vi "get_rumble_video_data.vi"(0 "HTTP client handle":T1, 1 "Private IDs (F)":bool, 3 "Embed delta":refnum<queue>, 5 "Video ID":cluster{"Index":i32, "Canonical ID":i32}, 7 "Thumbnails folder":path, 11 "error in (no error)":errorcluster, 12 "Rate limit ref.":refnum<vi>, 14 "Result queue":refnum<queue>) -> (4 "client handle out":T1, 15 "error out":errorcluster)   [LabVIEW 2023]
uses:
  <vilib>/httpClient/ClientHandle.ctl
  <vilib>/httpClient/LabVIEWHTTPClient.lvlib
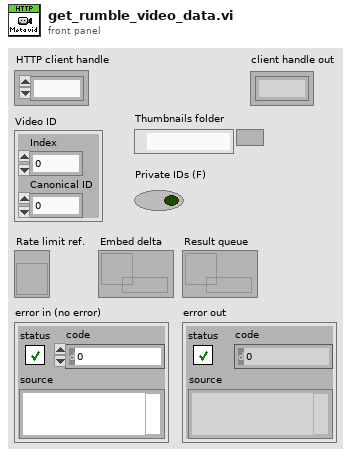
[diagram p1: front panel]
types:
  T1 = typedef "LabVIEWHTTPClient.lvlib/ClientHandle.ctl" = refnum<k1>
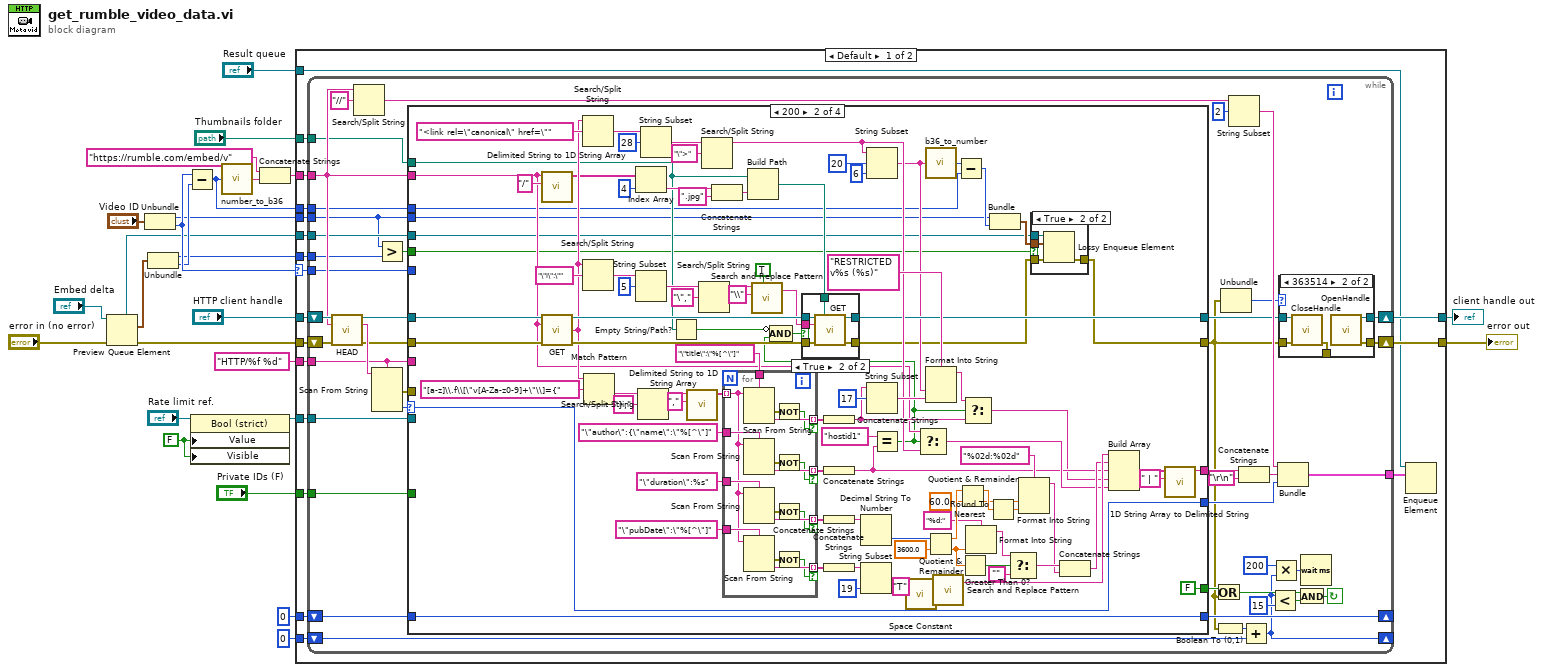
[diagram p0: block diagram]
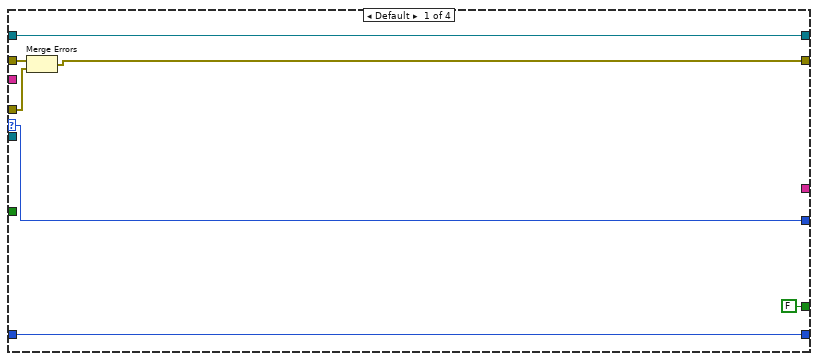
[diagram p3: hidden frame]
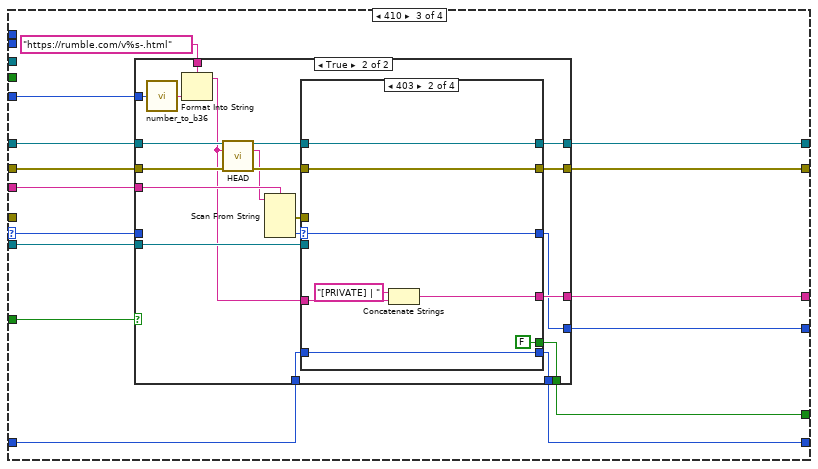
[diagram p6: hidden frame]
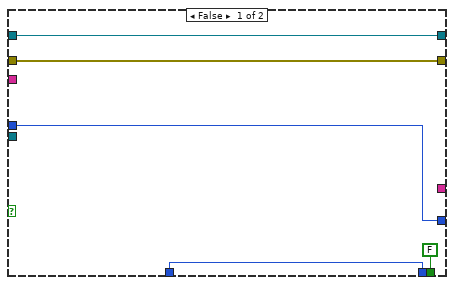
[diagram p7: hidden frame]
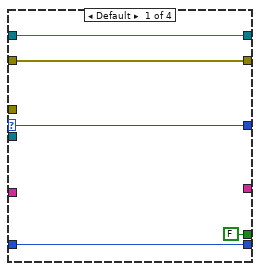
[diagram p8: hidden frame]
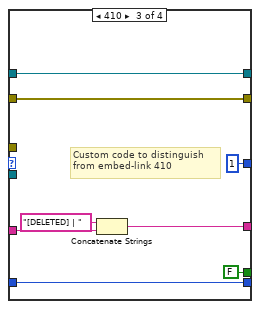
[diagram p9: hidden frame]
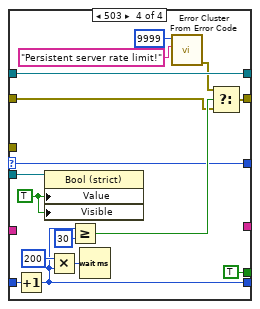
[diagram p10: hidden frame]
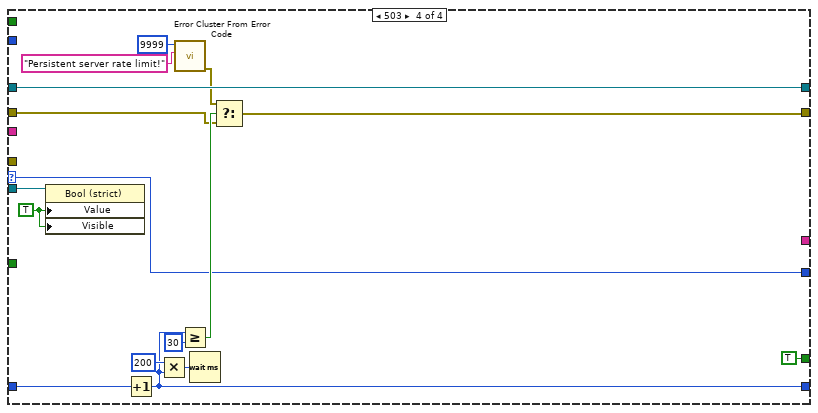
[diagram p11: hidden frame]
diagram:
  w18 = FALSE ("Value")
  n1 = Preview Queue Element(queue="Embed delta", error in (no error)="error in (no error)") -> (queue out=w4:refnum<queue>, element=w9:cluster{"Index":i32, "Embed delta":i32}, error out=w8:errorcluster)  [unwired: 1 in, 1 out]
  n2 = Unbundle("Video ID") -> ("Index"=w1:i32, "Canonical ID"=w7:i32)
  n3 = Unbundle(w9) -> ("Index"=w3:i32, "Embed delta"=w6:i32)
  n4 = Subtract(x=w7, y=w6) -> (x-y=w2:i32)
  n5 = property class="Bool (strict)"(reference="Rate limit ref.", "Value"=w18, "Visible"=w18) -> (reference out=w21:refnum<vi>)  [unwired: 1 in, 1 out]
  n6 = call "number_to_b36.vi"("Number"=w2) -> ("Base36 string"=w5:string)
  n7 = Concatenate Strings("https://rumble.com/embed/v" ("url"), w5) -> (w14:string)
  n8 = case shown="Default" w7 {
    selector: w7 -> [w31 _]
    tunnel: [w44 w324] -> w26
    tunnel: [w43 w323] -> w25
    tunnel: "HTTP client handle" -> [w42 w324]
    tunnel: w8 -> [w41 w323]
    tunnel: "HTTP/%f %d" ("format string") -> [w40 _]
    tunnel: w21 -> [w39 _]
    tunnel: 0 -> [w38 _]
    tunnel: 0 -> [w37 _]
    tunnel: w14 -> [w35 _]
    tunnel: "Thumbnails folder" -> [w34 _]
    tunnel: "Result queue" -> [w33 _]
    tunnel: "Private IDs (F)" -> [w32 _]
    tunnel: w4 -> [w30 _]
    tunnel: w1 -> [w29 _]
    tunnel: w3 -> [w28 _]
    tunnel: w2 -> [w27 _]
    frame Default {
      n9 = while {
        tunnel: w40 -> [w63]
        tunnel: w39 -> [w84]
        shift-right: [w52] -> w44
        shift-left: w42 -> [w88]
        shift-right: [w51] -> w43
        shift-left: w41 -> [w87]
        shift-right: [w59] -> _
        shift-left: w38 -> [w82]
        shift-right: [w79] -> _
        shift-left: w37 -> [w80]
        tunnel: w35 -> [w69]
        tunnel: [w70] -> w36
        tunnel: w34 -> [w65]
        tunnel: w31 -> [w64]
        tunnel: w32 -> [w50]
        tunnel: w30 -> [w49]
        tunnel: w29 -> [w48]
        tunnel: w28 -> [w46]
        tunnel: w27 -> [w47]
        stop <- w75 continue-if-true
        n10 = call <vilib>:"HEAD.vi"("client handle"=w88, "url"=w69, "error in (no error)"=w87) -> ("client handle out"=w85:T1, "headers"=w86:string, "error out"=w57:errorcluster)  [unwired: 10 in]
        n11 = Search/Split String(string=w69, search string/char (-)="//") -> (match + rest of string=w67:string)  [unwired: 1 in, 2 out]
        n12 = Scan From String(format string=w63, input string=w86) -> (error out=w72:errorcluster, output 2=w58:i32)  [unwired: 5 in, 2 out]
        n13 = Greater?(x=w48, y=w46) -> (0:w45:bool)
        n14 = case shown="200" w58 {
          selector: w58 -> [w96 w113 w234 w307]
          tunnel: [w102 w136 w240 w322] -> w54
          tunnel: [w97 w104 w239 w309] -> w53
          tunnel: w85 -> [w102 w152 w244 w322]
          tunnel: w57 -> [w99 w151 w243 w311]
          tunnel: w69 -> [_ w119 _ _]
          tunnel: [_ w155 w231 _] -> w73
          tunnel: w84 -> [_ _ w241 w321]
          tunnel: [FALSE FALSE w235 TRUE] -> w81
          tunnel: w80 -> [w100 w153 w238 w319]
          tunnel: [w100 w153 w237 w315] -> w79
          tunnel: w72 -> [w98 _ _ _]
          tunnel: w65 -> [_ w117 _ _]
          tunnel: w64 -> [_ _ w230 _]
          tunnel: w63 -> [_ _ w242 _]
          tunnel: [w96 w113 w236 w307] -> w62
          tunnel: w50 -> [_ _ w233 _]
          tunnel: w49 -> [_ w106 _ _]
          tunnel: w48 -> [_ w108 _ _]
          tunnel: w47 -> [_ w110 _ _]
          tunnel: w45 -> [_ w103 _ _]
          frame Default {
            n15 = Merge Errors(w99, w98) -> (w97:errorcluster)
          }
          frame 200 {
            n16 = call <vilib>:"Delimited String to 1D String Array.vi"("delimiter"="/", "delimited string"=w119) -> ("string array"=w124:string[])  [unwired: 9 in]
            n17 = call <vilib>:"GET.vi"("client handle"=w152, "url"=w119, "error in (no error)"=w151) -> ("client handle out"=w138:T1, "body"=w127:string, "error out"=w137:errorcluster)  [unwired: 9 in, 1 out]
            n18 = Search/Split String(string=w127, search string/char (-)="<link rel=\"canonical\" href=\"") -> (match + rest of string=w165:string)  [unwired: 1 in, 2 out]
            n19 = Search/Split String(string=w127, search string/char (-)="\"i\":\"") -> (match + rest of string=w129:string)  [unwired: 1 in, 2 out]
            n20 = Match Pattern(string=w127, regular expression="[a-z]\\.f\\[\"v[A-Za-z0-9]+\"\\]={") -> (after substring=w197:string)  [unwired: 1 in, 3 out]
            n21 = Index Array(array=w124, index=4) -> (element=w120:string)
            n22 = String Subset(string=w129, offset (0)=5) -> (substring=w132:string)  [unwired: 1 in]
            n23 = Search/Split String(string=w197, search string/char (-)="};") -> (substring before match=w196:string)  [unwired: 1 in, 2 out]
            n24 = String Subset(string=w165, offset (0)=28 ("y")) -> (substring=w168:string)  [unwired: 1 in]
            n25 = Empty String/Path?(string/path=w117) -> (empty?=w116:bool)
            n26 = call <vilib>:"Delimited String to 1D String Array.vi"("delimiter"=",", "delimited string"=w196) -> ("string array"=w194:string[])  [unwired: 9 in]
            n27 = Search/Split String(string=w132, search string/char (-)="\",") -> (substring before match=w133:string)  [unwired: 1 in, 2 out]
            n28 = Search/Split String(string=w168, search string/char (-)="\">") -> (substring before match=w139:string)  [unwired: 1 in, 2 out]
            n29 = Concatenate Strings(w120, ".jpg" ("string")) -> (w121:string)
            n30 = for {
              tunnel: w194 -> [w213] mode=indexing
              tunnel: "\"title\":\"%[^\"]" ("String") -> [w229]
              tunnel: "\"author\":{\"name\":\"%[^\"]" ("String") -> [w228]
              tunnel: "\"duration\":%s" ("String") -> [w227]
              tunnel: "\"pubDate\":\"%[^\"]" ("String") -> [w226]
              tunnel: [w225] -> w189 mode=indexing if=w217
              tunnel: [w224] -> w188 mode=indexing if=w216
              tunnel: [w223] -> w187 mode=indexing if=w215
              tunnel: [w222] -> w186 mode=indexing if=w214
              n31 = Scan From String(format string=w229, input string=w213) -> (error out=w221:errorcluster, output 1=w225:string)  [unwired: 3 in, 2 out]
              n32 = Scan From String(format string=w228, input string=w213) -> (error out=w220:errorcluster, output 1=w224:string)  [unwired: 3 in, 2 out]
              n33 = Scan From String(format string=w227, input string=w213) -> (error out=w219:errorcluster, output 1=w223:string)  [unwired: 3 in, 2 out]
              n34 = Scan From String(format string=w226, input string=w213) -> (error out=w218:errorcluster, output 1=w222:string)  [unwired: 3 in, 2 out]
              n35 = Not(x=w221) -> (.not. x?=w217:bool)
              n36 = Not(x=w220) -> (.not. x?=w216:bool)
              n37 = Not(x=w219) -> (.not. x?=w215:bool)
              n38 = Not(x=w218) -> (.not. x?=w214:bool)
            }
            n39 = Build Path(base path=w117, name or relative path=w121) -> (appended path=w118:path)
            n40 = call <vilib>:"Search and Replace Pattern.vi"("string"=w133, "regular expression (\"\")"="\\" ("regular expression (\"\")"), "replace all? (F)"=TRUE) -> ("result string"=w126:string)  [unwired: 2 in, 1 out]
            n41 = Concatenate Strings(w189) -> (w143:string)
            n42 = Concatenate Strings(w188) -> (w148:string)
            n43 = Concatenate Strings(w187) -> (w185:string)
            n44 = Concatenate Strings(w186) -> (w164:string)
            n45 = Decimal String To Number(string=w185) -> (number=w170:i32)  [unwired: 2 in, 1 out]
            n46 = String Subset(string=w164, length (rest)=19 ("length (rest)")) -> (substring=w162:string)  [unwired: 1 in]
            n47 = String Subset(string=w139, offset (0)=20 ("y"), length (rest)=6 ("length (rest)")) -> (substring=w112:string)
            n48 = String Subset(string=w143, offset (0)=17 ("y")) -> (substring=w145:string)  [unwired: 1 in]
            n49 = Equal?(x="hostid1", y=w148) -> (x = y?=w114:bool)
            n50 = Compound Arithmetic op=AND(invert w116, w114) -> (w115:bool)
            n51 = case shown="True" w115 {
              tunnel: w138 -> [w206 w212]
              tunnel: w137 -> [w205 w211]
              tunnel: [w206 w210] -> w136
              tunnel: [w205 w209] -> w105
              tunnel: w126 -> [_ w208]
              tunnel: w118 -> [_ w207]
              frame False {
              }
              frame True {
                n52 = call <vilib>:"GET.vi"("client handle"=w212, "output file"=w207, "url"=w208, "error in (no error)"=w211) -> ("client handle out"=w210:T1, "error out"=w209:errorcluster)  [unwired: 8 in, 2 out]
              }
            }
            n53 = call <vilib>:"Space Constant.vi"() -> ("String"=w160:string)
            n54 = Select(t=w119, s=w114, f=w139) -> (s? t:f=w149:string)
            n55 = call "b36_to_number.vi"("Base36 string"=w112) -> ("Number"=w111:i32)
            n56 = Format Into String(format string="RESTRICTED v%s (%s)", w112, w145) -> (resulting string=w144:string)  [unwired: 2 in, 1 out]
            n57 = Quotient & Remainder(x=w170, y=3600.0) -> (x-y*floor(x/y)=w183:dbl, floor(x/y)=w172:dbl)
            n58 = call <vilib>:"Search and Replace Pattern.vi"("string"=w162, "regular expression (\"\")"="T" ("regular expression (\"\")"), "replace string (\"\")"=w160) -> ("result string"=w159:string)  [unwired: 2 in, 1 out]
            n59 = Subtract(x=w111, y=w110) -> (x-y=w109:i32)
            n60 = Quotient & Remainder(x=w183, y=60.0) -> (x-y*floor(x/y)=w181:dbl, floor(x/y)=w176:dbl)
            n61 = Greater Than 0?(x=w172) -> (x > 0?=w180:bool)
            n62 = Select(t=w144, s=w114, f=w143) -> (s? t:f=w142:string)
            n63 = Format Into String(format string="%d:", w172) -> (resulting string=w171:string)  [unwired: 2 in, 1 out]
            n64 = Round To Nearest(number=w181) -> (nearest integer value=w175:dbl)
            n65 = Bundle("Index"=w108, w109) -> (w107:cluster{"Index":i32, i32})  [unwired: 1 in]
            n66 = Select(t=w171, s=w180, f="") -> (s? t:f=w178:string)
            n67 = Format Into String(format string="%02d:%02d", w176, w175) -> (resulting string=w174:string)  [unwired: 2 in, 1 out]
            n68 = case shown="True" w103 {
              tunnel: w107 -> [_ w204]
              tunnel: w106 -> [_ w203]
              tunnel: w105 -> [w200 w202]
              tunnel: [w200 w201] -> w104
              frame False {
              }
              frame True {
                n69 = Lossy Enqueue Element(queue=w203, element=w204, error in (no error)=w202) -> (error out=w201:errorcluster)  [unwired: 3 out]
              }
            }
            n70 = Concatenate Strings(w178, w174) -> (w158:string)
            n71 = Build Array(w159, w158, w148, w142, w149) -> (w157:string[])
            n72 = call <vilib>:"1D String Array to Delimited String.vi"("delimiter"=" | ", "string array"=w157) -> ("delimited string"=w155:string)  [unwired: 9 in]
          }
          frame 410 {
            n73 = case shown="True" w233 {
              tunnel: w244 -> [w245 w269]
              tunnel: w243 -> [w246 w268]
              tunnel: w242 -> [_ w267]
              tunnel: [_ w266] -> w231
              tunnel: w241 -> [_ w263]
              tunnel: [w245 w262] -> w240
              tunnel: [w246 w260] -> w239
              tunnel: w238 -> [w249 w258]
              tunnel: [w249 w257] -> w237
              tunnel: [w247 w253] -> w236
              tunnel: [FALSE w255] -> w235
              tunnel: w234 -> [w247 _]
              tunnel: "https://rumble.com/v%s-.html" ("url") -> [_ w254]
              tunnel: w230 -> [_ w251]
              frame False {
              }
              frame True {
                n74 = call "number_to_b36.vi"("Number"=w251) -> ("Base36 string"=w250:string)
                n75 = Format Into String(format string=w254, w250) -> (resulting string=w252:string)  [unwired: 2 in, 1 out]
                n76 = call <vilib>:"HEAD.vi"("client handle"=w269, "url"=w252, "error in (no error)"=w268) -> ("client handle out"=w261:T1, "headers"=w256:string, "error out"=w259:errorcluster)  [unwired: 10 in]
                n77 = Scan From String(format string=w267, input string=w256) -> (error out=w264:errorcluster, output 2=w265:i32)  [unwired: 5 in, 2 out]
                n78 = case shown="403" w265 {
                  selector: w265 -> [w271 w276 _ w292]
                  tunnel: [_ w280 w284 _] -> w266
                  tunnel: w252 -> [_ w281 w289 _]
                  tunnel: w264 -> [_ _ _ _]
                  tunnel: w263 -> [_ _ _ w305]
                  tunnel: [w274 w278 w287 w304] -> w262
                  tunnel: w261 -> [w274 w278 w287 w304]
                  tunnel: [w273 w279 w288 w294] -> w260
                  tunnel: w259 -> [w273 w279 w288 w295]
                  tunnel: w258 -> [w272 w277 w286 w300]
                  tunnel: [w272 w277 w286 w293] -> w257
                  tunnel: [w271 w276 1 w292] -> w253
                  tunnel: [FALSE FALSE FALSE TRUE] -> w255
                  frame Default {
                  }
                  frame 403 {
                    n79 = Concatenate Strings("[PRIVATE] | " ("format string"), w281) -> (w280:string)
                  }
                  frame 410 {
                    # "Custom code to distinguish\nfrom embed-link 410"
                    n80 = Concatenate Strings("[DELETED] | " ("format string"), w289) -> (w284:string)
                  }
                  frame 503 {
                    w306 = TRUE ("Value")
                    n81 = Increment(x=w300) -> (x+1=w293:i32)
                    n82 = property class="Bool (strict)"(reference=w305, "Value"=w306, "Visible"=w306) -> ()  [unwired: 1 in, 2 out]
                    n83 = Multiply(x=u32 200 ("milliseconds to wait"), y=w293) -> (x*y=w302:u32)
                    n84 = Greater Or Equal?(x=w293, y=30) -> (x >= y?=w296:bool)
                    n85 = Wait (ms)(milliseconds to wait=w302) -> ()  [unwired: 1 out]
                    n86 = call <vilib>:"Error Cluster From Error Code.vi"("error message (\"\")"="Persistent server rate limit!" ("error message (\"\")"), "error code (0)"=9999) -> ("error out"=w297:errorcluster)  [unwired: 7 in]
                    n87 = Select(t=w297, s=w296, f=w295) -> (s? t:f=w294:errorcluster)
                  }
                }
              }
            }
          }
          frame 503 {
            w308 = TRUE ("Value")
            n88 = property class="Bool (strict)"(reference=w321, "Value"=w308, "Visible"=w308) -> ()  [unwired: 1 in, 2 out]
            n89 = Increment(x=w319) -> (x+1=w315:i32)
            n90 = Multiply(x=u32 200 ("milliseconds to wait"), y=w315) -> (x*y=w317:u32)
            n91 = call <vilib>:"Error Cluster From Error Code.vi"("error message (\"\")"="Persistent server rate limit!" ("error message (\"\")"), "error code (0)"=9999) -> ("error out"=w310:errorcluster)  [unwired: 7 in]
            n92 = Greater Or Equal?(x=w315, y=30) -> (x >= y?=w312:bool)
            n93 = Wait (ms)(milliseconds to wait=w317) -> ()  [unwired: 1 out]
            n94 = Select(t=w310, s=w312, f=w311) -> (s? t:f=w309:errorcluster)
          }
        }
        n95 = Or(x=w81, y=w53) -> (x .or. y?=w76:bool)
        n96 = Boolean To (0,1)(Boolean=w53) -> (0, 1=w83:i16)
        n97 = Unbundle(w53) -> ("code"=w55:i32)  [unwired: 2 out]
        n98 = String Subset(string=w67, offset (0)=2) -> (substring=w56:string)  [unwired: 1 in]
        n99 = Concatenate Strings(w73, "\r\n") -> (w71:string)
        n100 = Add(x=w83, y=w82) -> (x+y=w59:i32)
        n101 = Less?(x=w59, y=15) -> (x < y?=w77:bool)
        n102 = Multiply(x=u32 200 ("milliseconds to wait"), y=w59) -> (x*y=w61:u32)
        n103 = Bundle(w56, w71, w62) -> (w70:cluster{string, string, i32})  [unwired: 1 in]
        n104 = case shown="363514" w55 {
          tunnel: w54 -> [w90 w95]
          tunnel: w53 -> [w89 w94]
          tunnel: [w90 w93] -> w52
          tunnel: [w89 w92] -> w51
          tunnel: [_ w91] -> _
          frame 0, Default {
          }
          frame 363514 {
            n105 = call <vilib>:"CloseHandle.vi"("client handle"=w95, "error in (no error)"=w94) -> ("error out"=w91:errorcluster)  [unwired: 13 in]
            n106 = call <vilib>:"OpenHandle.vi"() -> ("client handle out"=w93:T1, "error out"=w92:errorcluster)  [unwired: 14 in]
          }
        }
        n107 = And(x=w76, y=w77) -> (x .and. y?=w75:bool)
        n108 = Wait (ms)(milliseconds to wait=w61) -> ()  [unwired: 1 out]
      }
      n109 = Enqueue Element(queue=w33, element=w36) -> ()  [unwired: 2 in, 3 out]
    }
    frame ..0 {
    }
  }
  "client handle out" <- w26
  "error out" <- w25
